vi "niRFUtil TRC Waveform to Trace (real array).vi"(7 "Real Array":T2 min=0 max=127 format="%.2f") -> (8 "Measurement Trace":T1 format="%.2f")   [LabVIEW 2015, in "niRFUtil.lvlib"]
doc: "(c) Copyright 2006, National Instruments, Inc. This VI may not be duplicated, sold, or distributed without written consent from National Instruments."
uses:
  niRFUtil.lvlib
  Includes/niRFUtil INC Real Array.ctl
  Includes/niRFUtil INC Trace.ctl
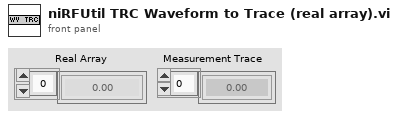
[diagram p1: front panel]
types:
  T1 = typedef "niRFUtil.lvlib/niRFUtil INC Trace.ctl" = sgl[]
  T2 = typedef "niRFUtil.lvlib/niRFUtil INC Real Array.ctl" = sgl[]
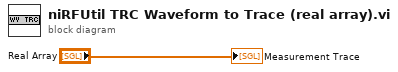
[diagram p0: block diagram]
diagram:
  "Measurement Trace" <- "Real Array"
